vi "ABAPI Dist Get Current VI Settings.vi"(11 "vi or ctl":T2) -> (3 "settings":T1)   [LabVIEW 2020]
uses:
  <vilib>/AppBuilder/ABAPI Dist VI Settings.ctl
panel:
  in  "use hints for keep panel? (T)":bool=TRUE
  # "T"
  # "F"
  # "F"
  # "F"
  # "F"
  # "F"
  # "T"
  # "T"
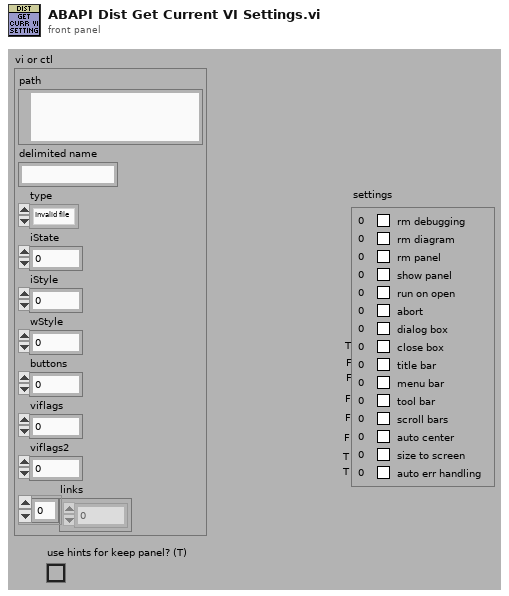
[diagram p1: front panel]
types:
  T1 = typedef "ABAPI Dist VI Settings.ctl" = cluster{"rm debugging":u16, "rm diagram":u16, "rm panel":u16, "show panel":u16, "run on open":u16, "abort":u16, "dialog box":u16, "close box":u16, "title bar":u16, "menu bar":u16, "tool bar":u16, "scroll bars":u16, "auto center":u16, "size to screen":u16, "auto err handling":u16}
  T2 = cluster{"path":path, "delimited name":string, "type":enum32{"Invalid file", "Unknown type", "Instrument", "Control", "Polymorphic VI", "Project", "Library", "LVClass", "XControl", "XNode", "Shared library", ".NET assembly", "ActiveX interface", "CIN", "Run-time menu", "Palette menu", "Help file", "LLB"}, "iState":u32, "iStyle":u16, "wStyle":u16, "buttons":u16, "viflags":u32, "viflags2":u32, "links":u32[]}
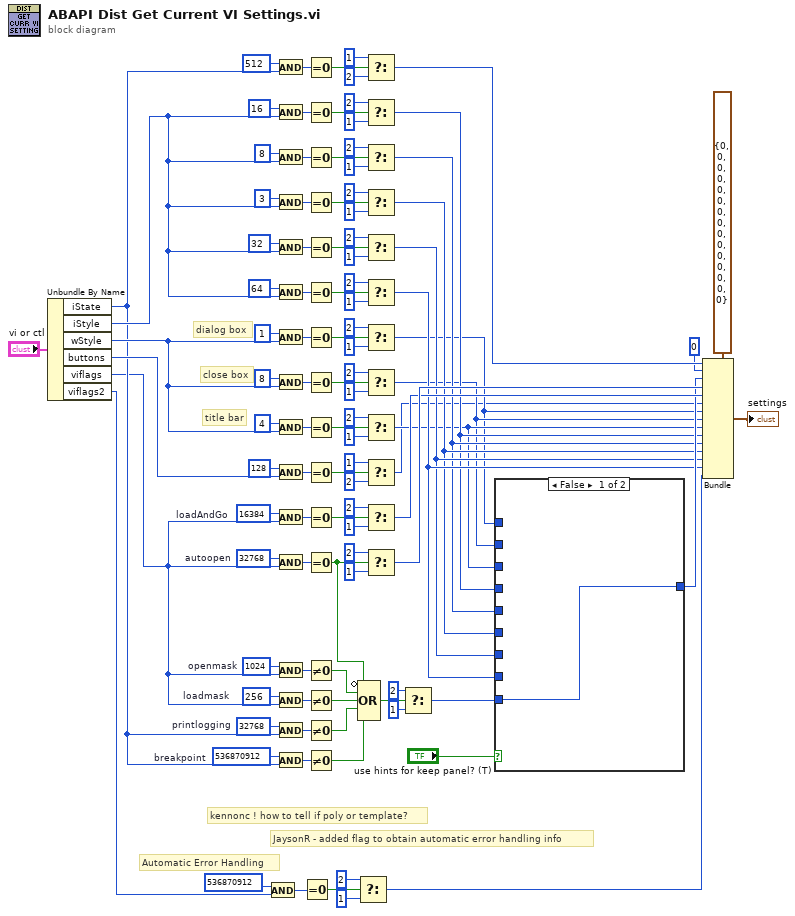
[diagram p0: block diagram]
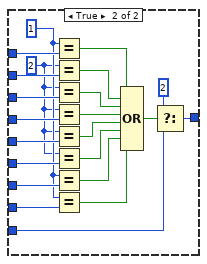
[diagram p2: hidden frame]
diagram:
  w26 = u32 16384  # loadAndGo
  w36 = u32 1024  # openmask
  w42 = u32 536870912  # breakpoint
  w44 = u32 32768  # printlogging
  w47 = u32 256  # loadmask
  w100 = u32 32768  # autoopen
  # "title bar"
  # "close box"
  # "dialog box"
  # "JaysonR - added flag to obtain automatic error handling info"
  # "Automatic Error Handling"
  # "kennonc ! how to tell if poly or template?"
  n1 = Unbundle By Name("vi or ctl") -> ("iState"=w39:u32, "iStyle"=w53:u16, "wStyle"=w75:u16, "buttons"=w86:u16, "viflags"=w20:u32, "viflags2"=w6:u32)
  n2 = And(x=u32 536870912, y=w6) -> (x .and. y?=w5:u32)
  n3 = And(x=u32 512, y=w39) -> (x .and. y?=w104:u32)
  n4 = And(x=u16 16, y=w53) -> (x .and. y?=w73:u16)
  n5 = And(x=u16 8, y=w53) -> (x .and. y?=w67:u16)
  n6 = And(x=u16 3, y=w53) -> (x .and. y?=w64:u16)
  n7 = And(x=u16 32, y=w53) -> (x .and. y?=w59:u16)
  n8 = And(x=u16 64, y=w53) -> (x .and. y?=w56:u16)
  n9 = And(x=u16 1, y=w75) -> (x .and. y?=w89:u16)
  n10 = And(x=u16 8, y=w75) -> (x .and. y?=w84:u16)
  n11 = And(x=u16 4, y=w75) -> (x .and. y?=w77:u16)
  n12 = And(x=u16 128, y=w86) -> (x .and. y?=w93:u16)
  n13 = And(x=w26, y=w20) -> (x .and. y?=w25:u32)
  n14 = And(x=w100, y=w20) -> (x .and. y?=w98:u32)
  n15 = And(x=w36, y=w20) -> (x .and. y?=w37:u32)
  n16 = And(x=w47, y=w20) -> (x .and. y?=w48:u32)
  n17 = And(x=w44, y=w39) -> (x .and. y?=w45:u32)
  n18 = And(x=w42, y=w39) -> (x .and. y?=w41:u32)
  n19 = Equal To 0?(x=w5) -> (x = 0?=w2:bool)
  n20 = Equal To 0?(x=w104) -> (x = 0?=w103:bool)
  n21 = Equal To 0?(x=w73) -> (x = 0?=w72:bool)
  n22 = Equal To 0?(x=w67) -> (x = 0?=w68:bool)
  n23 = Equal To 0?(x=w64) -> (x = 0?=w63:bool)
  n24 = Equal To 0?(x=w59) -> (x = 0?=w60:bool)
  n25 = Equal To 0?(x=w56) -> (x = 0?=w55:bool)
  n26 = Equal To 0?(x=w89) -> (x = 0?=w90:bool)
  n27 = Equal To 0?(x=w84) -> (x = 0?=w83:bool)
  n28 = Equal To 0?(x=w77) -> (x = 0?=w78:bool)
  n29 = Equal To 0?(x=w93) -> (x = 0?=w94:bool)
  n30 = Equal To 0?(x=w25) -> (x = 0?=w24:bool)
  n31 = Equal To 0?(x=w98) -> (x = 0?=w38:bool)
  n32 = Not Equal To 0?(x=w37) -> (x != 0?=w35:bool)
  n33 = Not Equal To 0?(x=w48) -> (x != 0?=w46:bool)
  n34 = Not Equal To 0?(x=w45) -> (x != 0?=w43:bool)
  n35 = Not Equal To 0?(x=w41) -> (x != 0?=w40:bool)
  n36 = Compound Arithmetic op=OR(invert w38, w35, w46, w43, w40) -> (w32:bool)
  n37 = Select(t=u16 2, s=w2, f=u16 1) -> (s? t:f=w1:u16)
  n38 = Select(t=u16 1, s=w103, f=u16 2) -> (s? t:f=w33:u16)
  n39 = Select(t=u16 2, s=w72, f=u16 1) -> (s? t:f=w13:u16)
  n40 = Select(t=u16 2, s=w68, f=u16 1) -> (s? t:f=w14:u16)
  n41 = Select(t=u16 2, s=w63, f=u16 1) -> (s? t:f=w15:u16)
  n42 = Select(t=u16 2, s=w60, f=u16 1) -> (s? t:f=w16:u16)
  n43 = Select(t=u16 2, s=w55, f=u16 1) -> (s? t:f=w17:u16)
  n44 = Select(t=u16 2, s=w90, f=u16 1) -> (s? t:f=w10:u16)
  n45 = Select(t=u16 2, s=w83, f=u16 1) -> (s? t:f=w11:u16)
  n46 = Select(t=u16 2, s=w78, f=u16 1) -> (s? t:f=w12:u16)
  n47 = Select(t=u16 1, s=w94, f=u16 2) -> (s? t:f=w9:u16)
  n48 = Select(t=u16 2, s=w24, f=u16 1) -> (s? t:f=w21:u16)
  n49 = Select(t=u16 2, s=w38, f=u16 1) -> (s? t:f=w97:u16)
  n50 = Select(t=u16 2, s=w32, f=u16 1) -> (s? t:f=w31:u16)
  n51 = case shown="False" "use hints for keep panel? (T)" {
    tunnel: w31 -> [w107 w111]
    tunnel: [w107 w113] -> w18
    tunnel: w17 -> [_ w122]
    tunnel: w16 -> [_ w123]
    tunnel: w15 -> [_ w124]
    tunnel: w14 -> [_ w125]
    tunnel: w13 -> [_ w126]
    tunnel: w12 -> [_ w127]
    tunnel: w11 -> [_ w128]
    tunnel: w10 -> [_ w129]
    frame False {
    }
    frame True {
      w120 = u16 2
      w121 = u16 1
      n52 = Equal?(x=w121, y=w129) -> (x = y?=w109:bool)
      n53 = Equal?(x=w120, y=w128) -> (x = y?=w119:bool)
      n54 = Equal?(x=w120, y=w127) -> (x = y?=w118:bool)
      n55 = Equal?(x=w120, y=w126) -> (x = y?=w117:bool)
      n56 = Equal?(x=w120, y=w125) -> (x = y?=w116:bool)
      n57 = Equal?(x=w120, y=w124) -> (x = y?=w115:bool)
      n58 = Equal?(x=w121, y=w123) -> (x = y?=w114:bool)
      n59 = Equal?(x=w121, y=w122) -> (x = y?=w108:bool)
      n60 = Compound Arithmetic op=OR(w109, w119, w118, w117, w116, w115, w114, w108) -> (w110:bool)
      n61 = Select(t=u16 2, s=w110, f=w111) -> (s? t:f=w113:u16)
    }
  }
  n62 = Bundle(cluster=T1 {"rm debugging"=0, "rm diagram"=0, "rm panel"=0, "show panel"=0, "run on open"=0, "abort"=0, "dialog box"=0, "close box"=0, "title bar"=0, "menu bar"=0, "tool bar"=0, "scroll bars"=0, "auto center"=0, "size to screen"=0, "auto err handling"=0} ("settings"), "rm debugging"=w33, "rm diagram"=u16 0, "rm panel"=w18, "show panel"=w97, "run on open"=w21, "abort"=w9, "dialog box"=w10, "close box"=w11, "title bar"=w12, "menu bar"=w13, "tool bar"=w14, "scroll bars"=w15, "auto center"=w16, "size to screen"=w17, "auto err handling"=w1) -> (→"settings":T1)
